vi "J1939 - Tool.vi"() -> ()   [LabVIEW 2019, in "J1939 Workspace Tool.lvlib"]
uses:
  J1939 Workspace Tool.lvlib
  NationalInstruments.VeriStand.SystemStorage
  Workspace Shared/Types/UI.StateVariables.ctl
  <vilib>/NI VeriStand/Display Template Support/DisplayTemplateSupport.llb/enum_Display Template Handler Minimal To Widget Msg.ctl
  <vilib>/NI VeriStand/Execution/Workspace/SystemStateRegEventRef.ctl
  <vilib>/NI VeriStand/Execution/Workspace/Target State Info.ctl
  <vilib>/NI VeriStand/Execution/Workspace/Target State.ctl
  Shared/Types/Private Data.ctl
  <vilib>/NI/STM/TCP/TCP Connection Info.ctl
  <vilib>/NI/STM/SubVIs/MetaDataElement.ctl
  Shared/Types/Error Cluster.ctl
  Shared/Types/Error Types.ctl
  <vilib>/NI VeriStand/Display Template Support/DisplayTemplateSupport.llb/enum_Display Template Handler Minimal To Workspace.ctl
  <vilib>/NI VeriStand/Execution/Workspace/WorkspaceAPI.ctl
  <vilib>/NI VeriStand/Execution/Workspace/SystemStateEventRef.ctl
  Workspace Shared/Types/UI.Refs.ctl
  <vilib>/Utility/miscctls.llb/LVStringsAndValuesArrayTypeDef_U8.ctl
  Shared/J1939 Utilities/SubVIs/Convert CAN Arb ID to J1939 ID.vi
  Shared/J1939 Utilities/J1939 Utilities.lvlib
  Shared/J1939 Addon Shared.lvlib
  <vilib>/NI/STM/NI STM.lvlib
  Workspace Shared/J1939 Workspace Shared.lvlib
  <vilib>/NI VeriStand/Execution/Workspace/NI_VS Workspace ExecutionAPI.lvlib
  NationalInstruments.VeriStand.ClientAPI
panel:
  in  "NIVS.Workspace Event":refnum<event-registration>
  in  "NIVS.Gateway IP Address":string
  in  "NIVS.System Definition Root":refnum<k24>
  in  "Tab Control":enum32{"DTCs", "Custom RQST", "RAW FRAME"}(tab)
  in  "Refresh Continuous":bool
  in  "Clear DTC":bool
  in  "Refresh DTCs":bool
  in  "DTCs":i32(listbox)
  in  "Addresses":string(tree)
  in  "Refresh Addresses":bool
  out "Response":string
  in  "Request":bool
  in  "PGN":u32 format="%.0x"
  in  "DA":u8(ring)
  in  "Clear Array":bool
  in  "RAW":bool
  out "Priority":u8 format="%02x"
  out "SA":u8 format="%02x"
  out "PGN":u32 format="%06x"
  in  "Identifier":u32 format="%08x"
  in  "Data":u8[](array[numeric])=[0, 0, 0, 0, 0, 0, 0, 0] format="%.0x"
  out "Device":string
  in  "Errors":bool
  # "This is the root reference to the active System Definition file. You could use this to read the configuration or populate a tree with channels. You are free to close this reference, but it will be closed for you if you don't."
  # "The SystemStorageUI .NET assembly provides controls to display data configured in the System Definition file."
  # "This is the IP Address of the VeriStand Gateway to which the Workspace is connected. Use this to open all the .NET Manager references. Usually the Gateway is running on localhost, but it could be running on a neighbor's machine."
  # "This registered string User Event is used to help instruct your tool to shut down when the Workspace is closing."
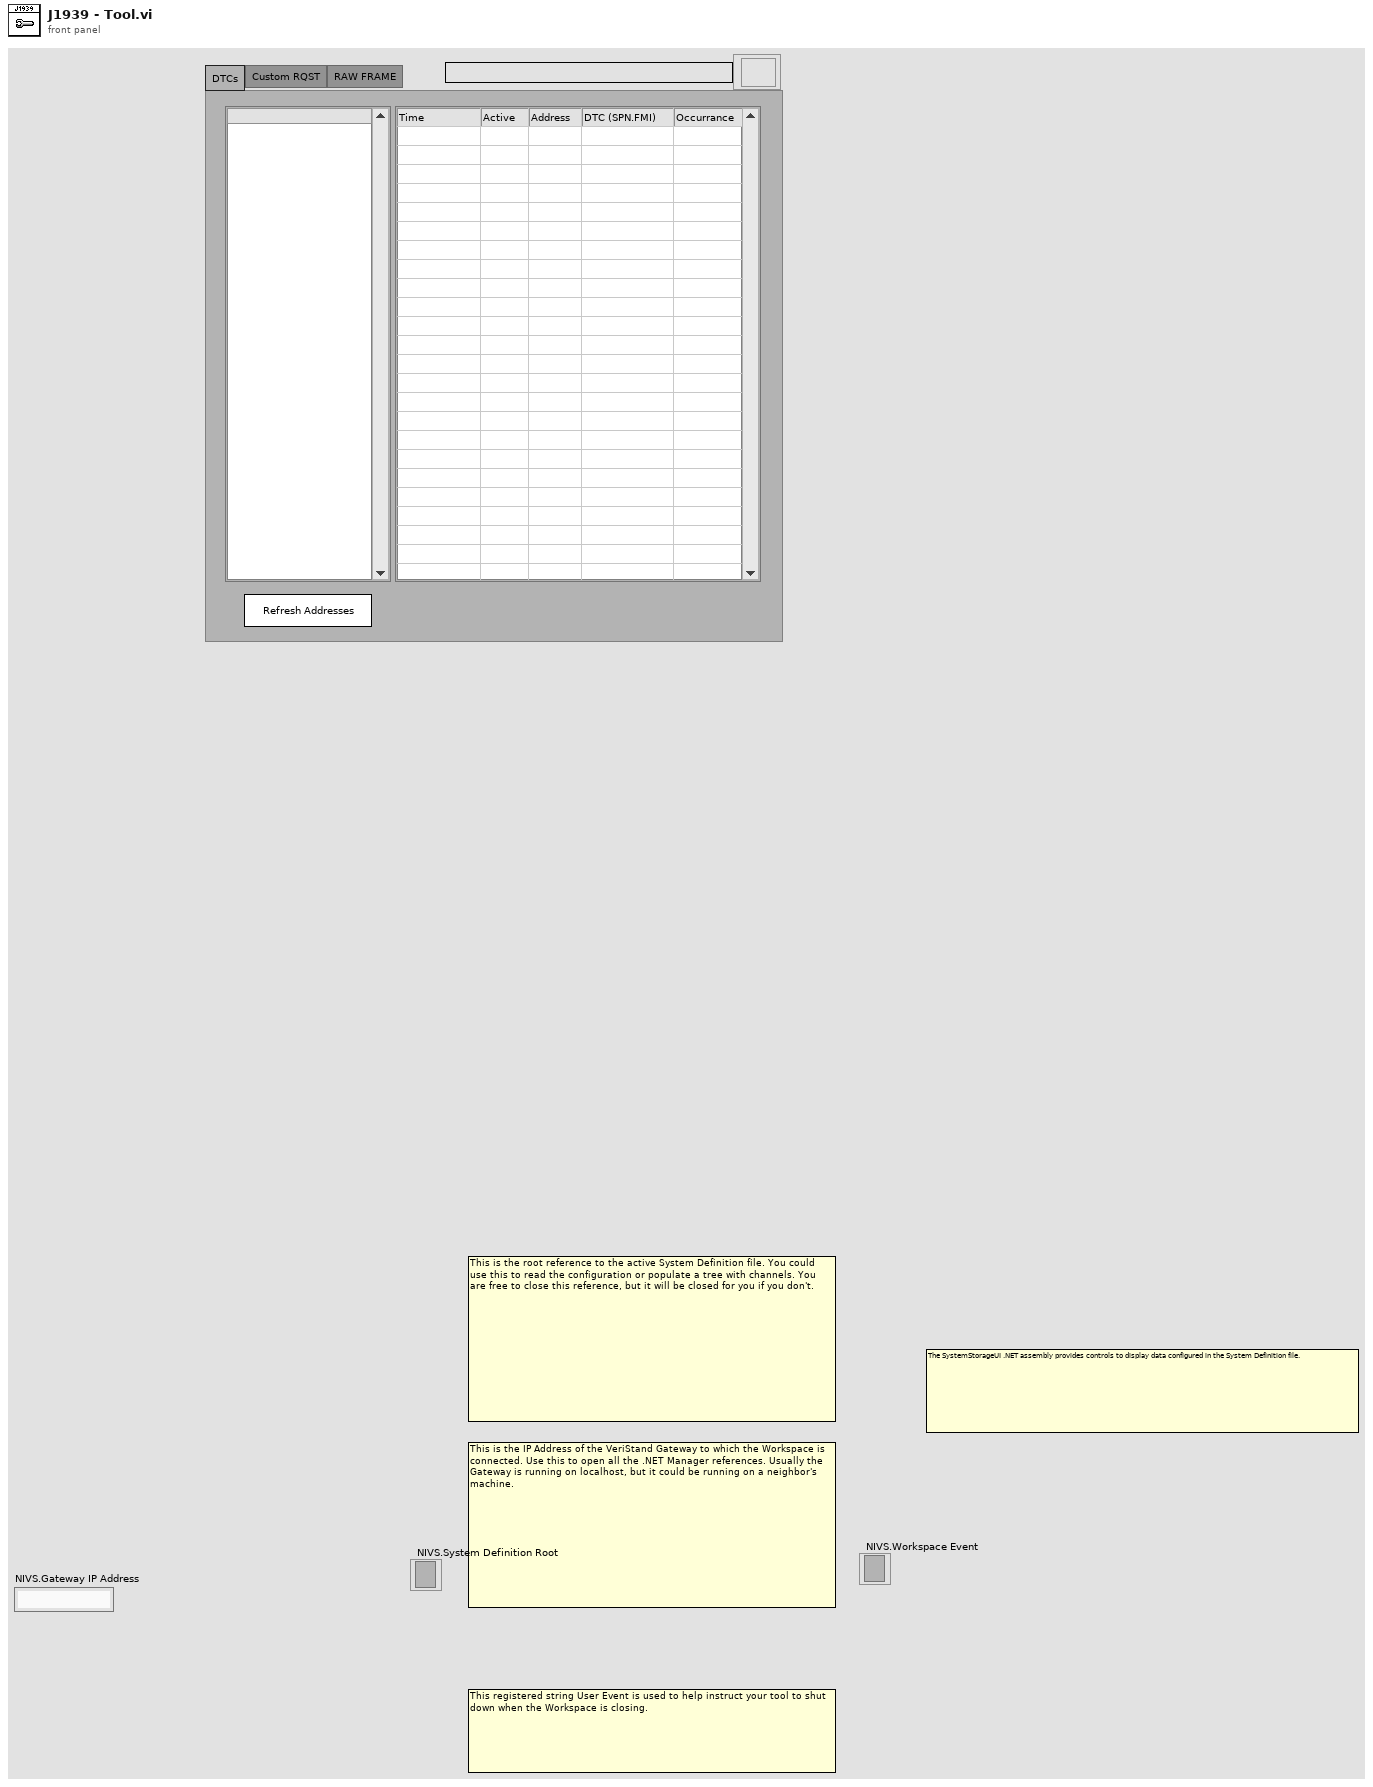
[diagram p1: front panel]
types:
  T1 = typedef "J1939 Addon Shared.lvlib/Private Data.ctl" = cluster{"PGN":u32, "DA":u8, "CD Path":string, "CD IP":string}
  T2 = typedef "J1939 Workspace Shared.lvlib/UI.StateVariables.ctl" = cluster{"NIVS.Gateway IP Address":string, "LaunchConfig.Ref":refnum<user-event>, "Events.Refs":cluster{"LaunchConfig":refnum<event-registration>, "SystemChange":T3, "NIVS.Workspace":refnum<event-registration>}, "State":T1, "TCP.Refs":T4, "Addresses.LUT":variant, "Errors.Q":refnum<queue>, "NIVS.SysDefRoot":refnum<k24>, "State.Notifier":refnum<user-event>, "NIVS.Workspace":T6, "DTCs.Refresh":bool, "NIVS.State.Refs":T7, "UI.Refs":T8, "Addon.Connected":bool, "DTCs.Timer":u32, "Mode.Tool?":bool}
  T3 = typedef "NI_VS Workspace ExecutionAPI.lvlib/SystemStateRegEventRef.ctl" = refnum<event-registration>
  T4 = typedef "NI STM.lvlib/TCP Connection Info.ctl" = cluster{"connection ID":refnum<k5>, "meta data":T5[]}
  T5 = typedef "NI STM.lvlib/MetaDataElement.ctl" = string
  T6 = typedef "NI_VS Workspace ExecutionAPI.lvlib/WorkspaceAPI.ctl" = refnum<k24>
  T7 = typedef "NI_VS Workspace ExecutionAPI.lvlib/SystemStateEventRef.ctl" = cluster{"CustDatRef":refnum<user-event>, "EvtRef":refnum<k27>, "Target State User Event":refnum<user-event>}
  T8 = typedef "J1939 Workspace Shared.lvlib/UI.Refs.ctl" = cluster{"ParentVI":refnum<vi>, "DTCs":refnum<vi>, "Addresses":refnum<vi>, "Device":refnum<vi>, "Data":refnum<vi>, "Identifier":refnum<vi>, "PGN":refnum<vi>, "DA":refnum<vi>, "Refresh Continuous":refnum<vi>, "Errors":refnum<vi>, "Refresh Addresses":refnum<vi>, "Refresh DTCs":refnum<vi>, "Clear DTC":refnum<vi>, "Request":refnum<vi>, "Clear Array":refnum<vi>, "RAW":refnum<vi>, "SA":refnum<vi>, "PGN Ind":refnum<vi>, "Priority":refnum<vi>, "Response":refnum<vi>}
  T9 = enum8{"Enabled", "Disabled", "Disabled and Grayed Out"}
  T10 = typedef "LVStringsAndValuesArrayTypeDef_U8.ctl" = cluster{"String":string, "Value":u8}[]
  T11 = typedef "enum_Display Template Handler Minimal To Workspace.ctl" = cluster{"Operation":enum16{"SetCustomData", "DeleteItem"}, "Data":variant}
  T12 = cluster{"LaunchConfig":refnum<event-registration>, "SystemChange":T3, "NIVS.Workspace":refnum<event-registration>}
  T13 = typedef "enum_Display Template Handler Minimal To Widget Msg.ctl" = enum16{"Stop", "LaunchConfigDialog"}
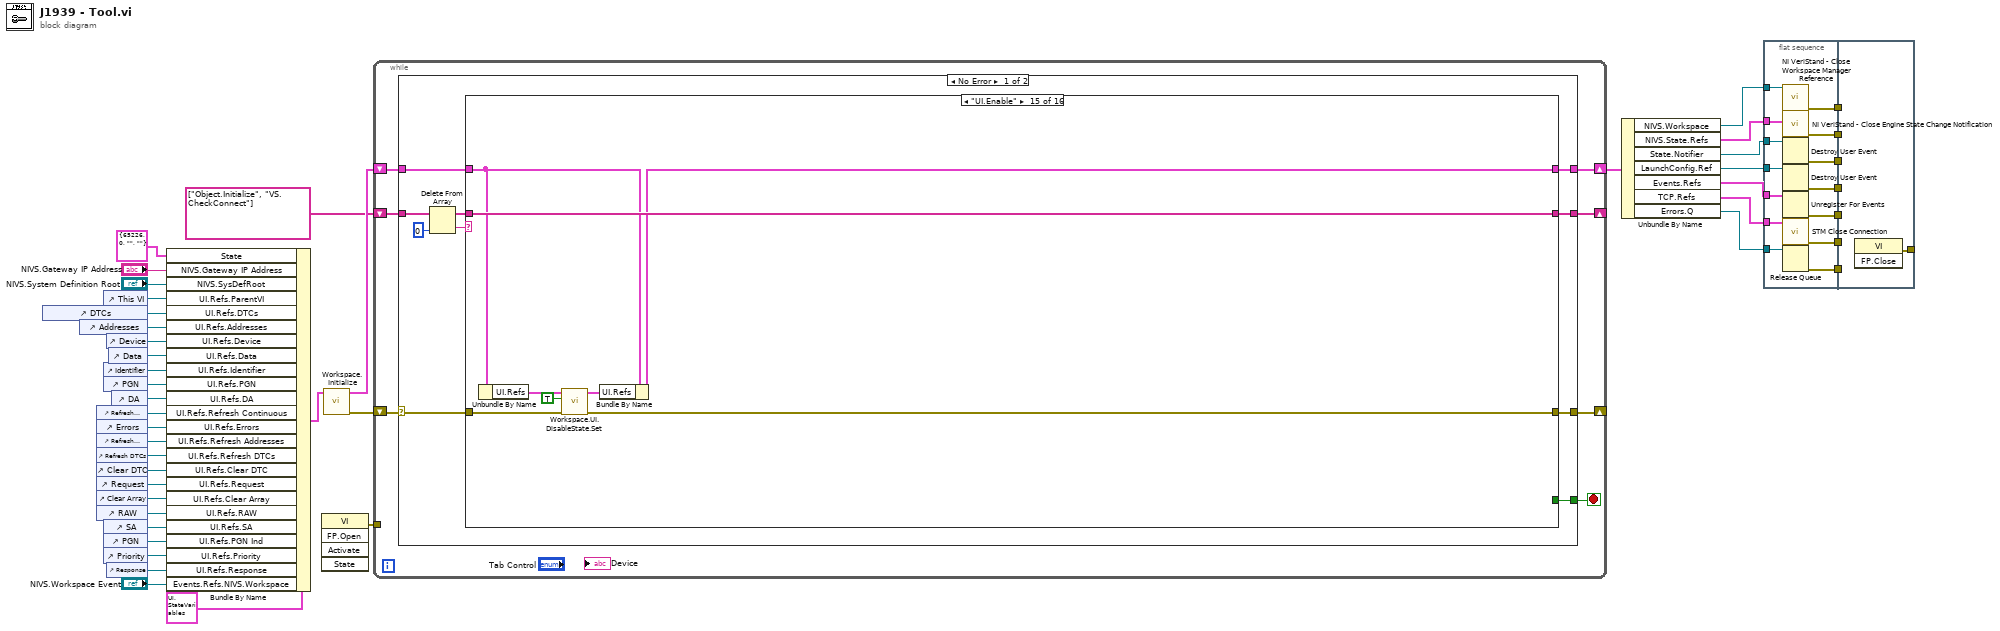
[diagram p0: block diagram]
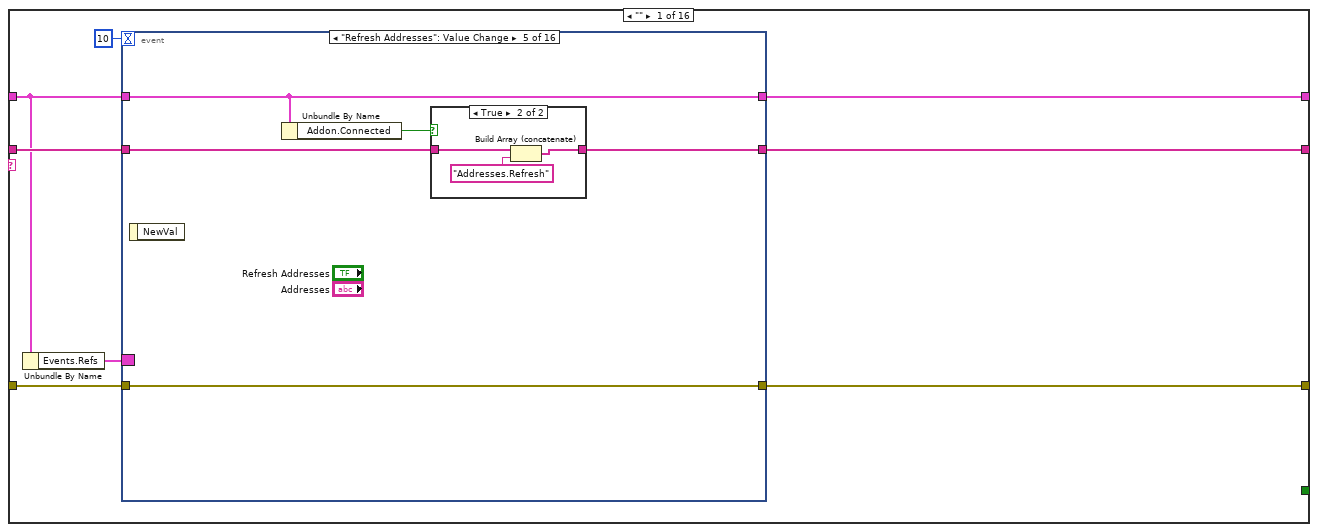
[diagram p2: hidden frame]
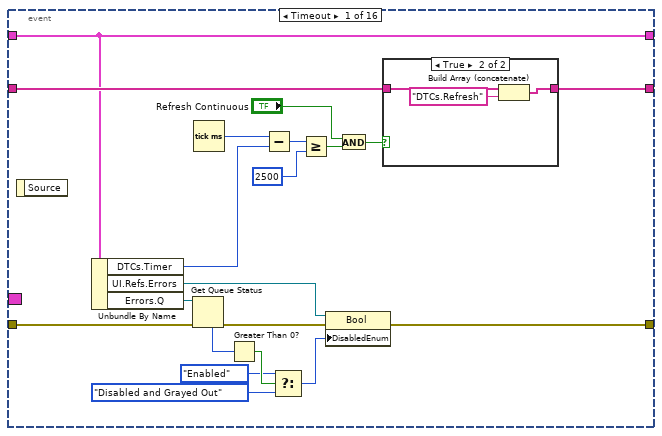
[diagram p3: hidden frame]
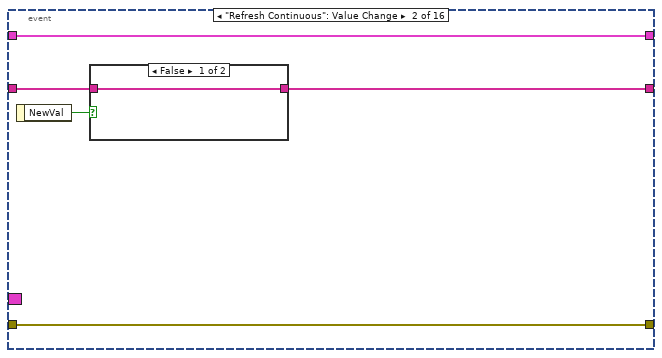
[diagram p5: hidden frame]
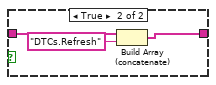
[diagram p6: hidden frame]
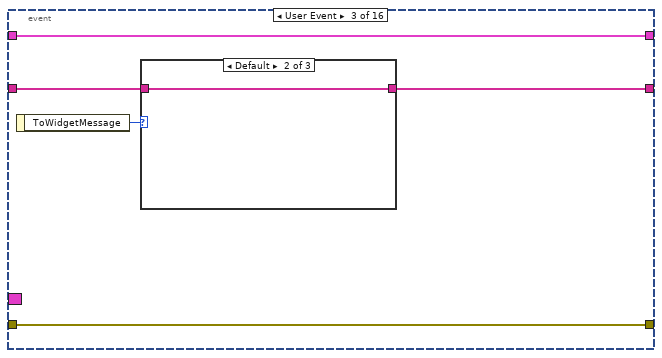
[diagram p7: hidden frame]
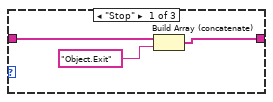
[diagram p8: hidden frame]
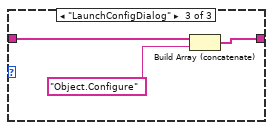
[diagram p9: hidden frame]
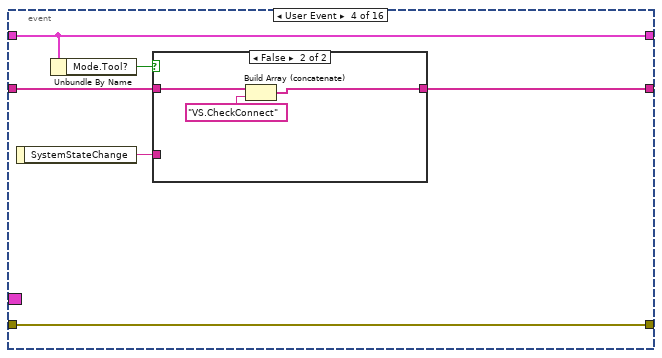
[diagram p10: hidden frame]
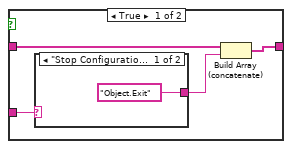
[diagram p11: hidden frame]
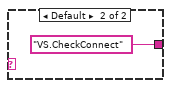
[diagram p12: hidden frame]
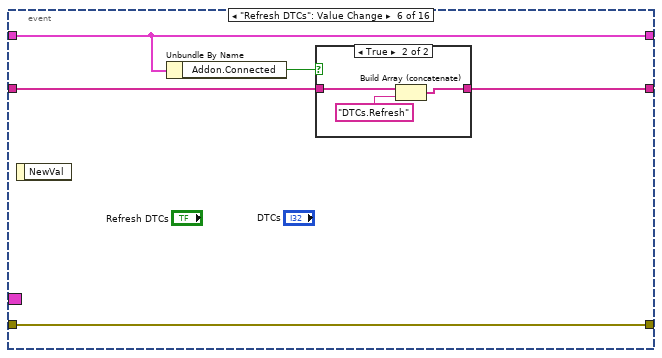
[diagram p14: hidden frame]
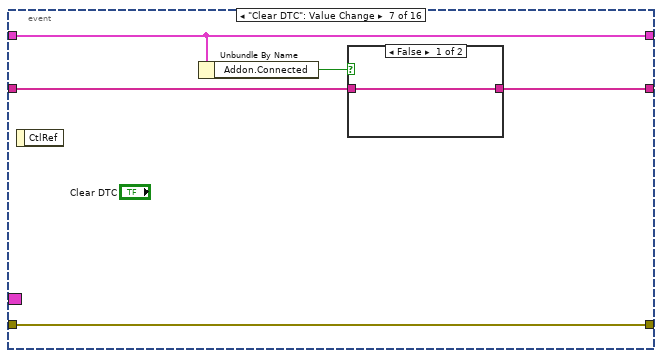
[diagram p16: hidden frame]
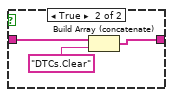
[diagram p17: hidden frame]
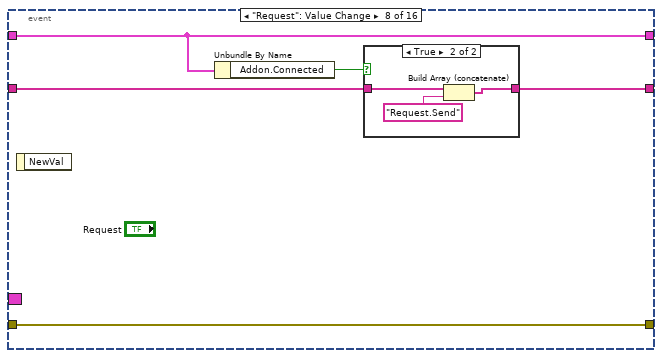
[diagram p18: hidden frame]
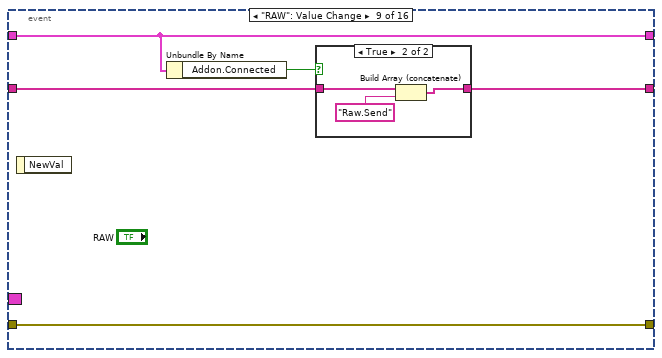
[diagram p20: hidden frame]
diagram:
  n1 = control-ref of="DTCs"() -> (w39:refnum<vi>)
  n2 = control-ref of="Addresses"() -> (w38:refnum<vi>)
  n3 = control-ref of="Refresh Continuous"() -> (w32:refnum<vi>)
  n4 = control-ref of="Errors"() -> (w31:refnum<vi>)
  n5 = control-ref of="Refresh Addresses"() -> (w30:refnum<vi>)
  n6 = control-ref of="Refresh DTCs"() -> (w29:refnum<vi>)
  n7 = control-ref of="Clear DTC"() -> (w28:refnum<vi>)
  n8 = control-ref of="Request"() -> (w27:refnum<vi>)
  n9 = control-ref of="Clear Array"() -> (w26:refnum<vi>)
  n10 = control-ref of="RAW"() -> (w25:refnum<vi>)
  n11 = control-ref of="This VI"() -> (w40:refnum<vi>)
  n12 = control-ref of="Identifier"() -> (w35:refnum<vi>)
  n13 = control-ref of="PGN"() -> (w34:refnum<vi>)
  n14 = control-ref of="SA"() -> (w4:refnum<vi>)
  n15 = control-ref of="PGN"() -> (w3:refnum<vi>)
  n16 = control-ref of="Priority"() -> (w2:refnum<vi>)
  n17 = control-ref of="Device"() -> (w37:refnum<vi>)
  n18 = control-ref of="Response"() -> (w1:refnum<vi>)
  n19 = control-ref of="Data"() -> (w36:refnum<vi>)
  n20 = control-ref of="DA"() -> (w33:refnum<vi>)
  n21 = Bundle By Name(cluster=T2 {"NIVS.Gateway IP Address"="", "LaunchConfig.Ref"=refnum, "Events.Refs"={"LaunchConfig"=refnum, "SystemChange"=refnum, "NIVS.Workspace"=refnum}, "State"={"PGN"=0, "DA"=0, "CD Path"="", "CD IP"=""}, "TCP.Refs"={"connection ID"=refnum, "meta data"=[]}, "Addresses.LUT"=variant, "Errors.Q"=refnum, "NIVS.SysDefRoot"=refnum, "State.Notifier"=refnum, "NIVS.Workspace"=refnum, "DTCs.Refresh"=FALSE, "NIVS.State.Refs"={"CustDatRef"=refnum, "EvtRef"=refnum, "Target State User Event"=refnum}, "UI.Refs"={"ParentVI"=refnum, "DTCs"=refnum, "Addresses"=refnum, "Device"=refnum, "Data"=refnum, "Identifier"=refnum, "PGN"=refnum, "DA"=refnum, "Refresh Continuous"=refnum, "Errors"=refnum, "Refresh Addresses"=refnum, "Refresh DTCs"=refnum, "Clear DTC"=refnum, "Request"=refnum, "Clear Array"=refnum, "RAW"=refnum, "SA"=refnum, "PGN Ind"=refnum, "Priority"=refnum, "Response"=refnum}, "Addon.Connected"=FALSE, "DTCs.Timer"=0, "Mode.Tool?"=FALSE}, "State"=T1 {"PGN"=65226, "DA"=0, "CD Path"="", "CD IP"=""} ("Cluster"), "NIVS.Gateway IP Address"="NIVS.Gateway IP Address", "NIVS.SysDefRoot"="NIVS.System Definition Root", "UI.Refs.ParentVI"=w40, "UI.Refs.DTCs"=w39, "UI.Refs.Addresses"=w38, "UI.Refs.Device"=w37, "UI.Refs.Data"=w36, "UI.Refs.Identifier"=w35, "UI.Refs.PGN"=w34, "UI.Refs.DA"=w33, "UI.Refs.Refresh Continuous"=w32, "UI.Refs.Errors"=w31, "UI.Refs.Refresh Addresses"=w30, "UI.Refs.Refresh DTCs"=w29, "UI.Refs.Clear DTC"=w28, "UI.Refs.Request"=w27, "UI.Refs.Clear Array"=w26, "UI.Refs.RAW"=w25, "UI.Refs.SA"=w4, "UI.Refs.PGN Ind"=w3, "UI.Refs.Priority"=w2, "UI.Refs.Response"=w1, "Events.Refs.NIVS.Workspace"="NIVS.Workspace Event") -> (w42:T2)
  n22 = invoke class="VI" method="FP.Open"() -> (error out=w12:errorcluster)  [unwired: 5 in, 4 out]
  n23 = call "Workspace.Initialize.vi"("State"=w42) -> ("error out"=w41:errorcluster, "State"=w24:T2)  [unwired: 9 in]
  n24 = while {
    shift-right: [w50] -> _
    shift-left: w41 -> [w51]
    shift-right: [w46] -> w22
    shift-left: w24 -> [w49]
    shift-right: [w47] -> _
    shift-left: string[] ["Object.Initialize", "VS.CheckConnect"] -> [w48]
    tunnel: w12 -> [_]
    stop <- w52 stop-if-true
    n25 = case shown="No Error" w51 {
      selector: w51 -> [w53 w461]
      tunnel: [w62 FALSE] -> w52
      tunnel: [w54 w459] -> w50
      tunnel: w49 -> [w61 w456]
      tunnel: w48 -> [w59 w457]
      tunnel: [w56 w457] -> w47
      tunnel: [w55 w456] -> w46
      frame No Error {
        n26 = Delete From Array(array=w59, index=0) -> (deleted portion=w58:string, array with subset deleted=w57:string[])  [unwired: 1 in]
        n27 = case shown="\"UI.Enable\"" w58 {
          selector: w58 -> [_ _ _ _ _ _ _ _ _ _ _ _ _ _ _ w451]
          tunnel: [_ _ _ _ _ _ _ _ TRUE _ _ _ _ _ _ _] -> w62
          tunnel: w61 -> [w64 w227 w236 w253 w306 w311 w345 w373 w376 w381 w405 w413 w425 w434 w442 w454]
          tunnel: w57 -> [w68 w234 w246 w262 w307 w309 w351 w369 w377 w379 w406 w414 w421 w441 w449 w455]
          tunnel: [w69 w234 w246 w262 w307 w308 w350 w369 w377 w378 w406 w414 w421 w441 w449 w455] -> w56
          tunnel: [w67 w224 w235 w263 w306 w310 w344 w372 w376 w382 w405 w412 w422 w435 w443 w454] -> w55
          tunnel: [w66 w223 w245 w248 w283 w314 w347 w368 w375 w390 w401 w407 w420 w436 w444 w453] -> w54
          tunnel: w53 -> [w65 w223 w245 w249 w280 w315 w346 w368 w375 w391 w400 w407 w420 w437 w445 w453]
          frame "" {
            n28 = Unbundle By Name(w64) -> ("Events.Refs"=w63:T12)
            n29 = event shown="[4] \"Refresh Addresses\": Value Change" {
              selector: w63 -> [_ _ _ _ _ _ _ _ _ _ _ _ _ _ _ _]
              dyn-events: _ -> [_ _ _ _ _ _ _ _ _ _ _ _ _ _ _ _]
              timeout: 10 -> [_ _ _ _ _ _ _ _ _ _ _ _ _ _ _ _]
              tunnel: w64 -> [w79 w98 w108 w117 w134 w142 w149 w160 w169 w178 w187 w191 w198 w208 w213 w222]
              tunnel: [w80 w96 w104 w120 w132 w140 w150 w158 w167 w176 w186 w192 w200 w204 w210 w219] -> w69
              tunnel: w68 -> [w81 w97 w105 w121 w133 w141 w151 w159 w168 w177 w189 w192 w200 w205 w211 w220]
              tunnel: [w79 w98 w108 w117 w134 w142 w149 w160 w169 w178 w187 w191 w198 w208 w213 w222] -> w67
              tunnel: [w73 w99 w107 w118 w135 w144 w153 w162 w171 w180 w188 w190 w199 w207 w212 w221] -> w66
              tunnel: w65 -> [w75 w99 w107 w118 w135 w144 w153 w162 w171 w180 w188 w190 w199 w207 w212 w221]
              event Timeout {
                n30 = event-data() -> ()  [unwired: 2 out]
                n31 = Unbundle By Name(w79) -> ("DTCs.Timer"=w72:u32, "UI.Refs.Errors"=w77:refnum<vi>, "Errors.Q"=w78:refnum<queue>)
                n32 = Get Queue Status(queue=w78, error in (no error)=w75) -> (error out=w76:errorcluster, # elements in queue=w90:i32)  [unwired: 1 in, 6 out]
                n33 = Tick Count (ms)() -> (millisecond timer value=w84:u32)
                n34 = Greater Than 0?(x=w90) -> (x > 0?=w89:bool)
                n35 = Subtract(x=w84, y=w72) -> (x-y=w86:u32)
                n36 = Select(t=T9."Enabled" ("Disabled"), s=w89, f=T9."Disabled and Grayed Out") -> (s? t:f=w74:T9)
                n37 = Greater Or Equal?(x=w86, y=u32 2500) -> (x >= y?=w71:bool)
                n38 = property class="Bool"(reference=w77, error in=w76, "DisabledEnum"=w74) -> (error out=w73:errorcluster)  [unwired: 1 out]
                n39 = And(x="Refresh Continuous", y=w71) -> (x .and. y?=w82:bool)
                n40 = case shown="True" w82 {
                  tunnel: w81 -> [w91 w93]
                  tunnel: [w91 w92] -> w80
                  frame False {
                  }
                  frame True {
                    n41 = Build Array (concatenate)(w93, "DTCs.Refresh" ("NewVal")) -> (w92:string[])
                  }
                }
              }
              event "Refresh Continuous": Value Change {
                n42 = event-data() -> ("NewVal"=w95:bool)  [unwired: 1 out]
                n43 = case shown="False" w95 {
                  tunnel: w97 -> [w100 w102]
                  tunnel: [w100 w101] -> w96
                  frame False {
                  }
                  frame True {
                    n44 = Build Array (concatenate)(w102, "DTCs.Refresh" ("NewVal")) -> (w101:string[])
                  }
                }
              }
              event User Event {
                n45 = event-data() -> ("ToWidgetMessage"=w106:T13)  [unwired: 1 out]
                n46 = case shown="Default" w106 {
                  tunnel: w105 -> [w111 w112 w115]
                  tunnel: [w110 w112 w114] -> w104
                  frame "Stop" {
                    n47 = Build Array (concatenate)(w111, "Object.Exit") -> (w110:string[])
                  }
                  frame Default {
                  }
                  frame "LaunchConfigDialog" {
                    n48 = Build Array (concatenate)(w115, "Object.Configure") -> (w114:string[])
                  }
                }
              }
              event User Event {
                n49 = event-data() -> ("SystemStateChange"=w116:string)  [unwired: 1 out]
                n50 = Unbundle By Name(w117) -> ("Mode.Tool?"=w119:bool)
                n51 = case shown="False" w119 {
                  tunnel: w121 -> [w125 w130]
                  tunnel: [w124 w129] -> w120
                  tunnel: w116 -> [w123 _]
                  frame True {
                    # "System state not connected"
                    n52 = case shown="\"Stop Configuration\"" w123 {
                      tunnel: ["Object.Exit" "VS.CheckConnect"] -> w122
                      frame "Stop Configuration" {
                      }
                      frame Default {
                      }
                    }
                    n53 = Build Array (concatenate)(w125, w122) -> (w124:string[])
                  }
                  frame False {
                    # "System state is connected"
                    n54 = Build Array (concatenate)(w130, "VS.CheckConnect") -> (w129:string[])
                  }
                }
              }
              event "Refresh Addresses": Value Change {
                n55 = event-data() -> ()  [unwired: 2 out]
                n56 = Unbundle By Name(w134) -> ("Addon.Connected"=w131:bool)
                n57 = case shown="True" w131 {
                  tunnel: w133 -> [w136 w138]
                  tunnel: [w136 w137] -> w132
                  frame False {
                  }
                  frame True {
                    n58 = Build Array (concatenate)(w138, "Addresses.Refresh") -> (w137:string[])
                  }
                }
              }
              event "Refresh DTCs": Value Change {
                n59 = event-data() -> ()  [unwired: 2 out]
                n60 = Unbundle By Name(w142) -> ("Addon.Connected"=w143:bool)
                n61 = case shown="True" w143 {
                  tunnel: w141 -> [w145 w147]
                  tunnel: [w145 w146] -> w140
                  frame False {
                  }
                  frame True {
                    n62 = Build Array (concatenate)(w147, "DTCs.Refresh") -> (w146:string[])
                  }
                }
              }
              event "Clear DTC": Value Change {
                n63 = event-data() -> ()  [unwired: 2 out]
                n64 = Unbundle By Name(w149) -> ("Addon.Connected"=w152:bool)
                n65 = case shown="False" w152 {
                  tunnel: w151 -> [w154 w156]
                  tunnel: [w154 w155] -> w150
                  frame False {
                  }
                  frame True {
                    n66 = Build Array (concatenate)(w156, "DTCs.Clear") -> (w155:string[])
                  }
                }
              }
              event "Request": Value Change {
                n67 = event-data() -> ()  [unwired: 2 out]
                n68 = Unbundle By Name(w160) -> ("Addon.Connected"=w161:bool)
                n69 = case shown="True" w161 {
                  tunnel: w159 -> [w163 w165]
                  tunnel: [w163 w164] -> w158
                  frame False {
                  }
                  frame True {
                    n70 = Build Array (concatenate)(w165, "Request.Send") -> (w164:string[])
                  }
                }
              }
              event "RAW": Value Change {
                n71 = event-data() -> ()  [unwired: 2 out]
                n72 = Unbundle By Name(w169) -> ("Addon.Connected"=w170:bool)
                n73 = case shown="True" w170 {
                  tunnel: w168 -> [w172 w174]
                  tunnel: [w172 w173] -> w167
                  frame False {
                  }
                  frame True {
                    n74 = Build Array (concatenate)(w174, "Raw.Send") -> (w173:string[])
                  }
                }
              }
              event "Clear Array": Value Change {
                n75 = event-data() -> ()  [unwired: 2 out]
                n76 = Unbundle By Name(w178) -> ("Addon.Connected"=w179:bool)
                n77 = case shown="True" w179 {
                  tunnel: w177 -> [w181 w183]
                  tunnel: [w181 w182] -> w176
                  frame False {
                  }
                  frame True {
                    n78 = Build Array (concatenate)(w183, "Raw.Clear") -> (w182:string[])
                  }
                }
              }
              event "Addresses": Value Change {
                n79 = event-data() -> ()  [unwired: 2 out]
                n80 = Build Array (concatenate)(w189, "DTCs.Refresh" ("NewVal")) -> (w186:string[])
              }
              event "Identifier": Value Change {
                n81 = event-data() -> ("NewVal"=w193:u32)  [unwired: 1 out]
                n82 = call-poly "Common Conversions.vi"("Arb ID"=w193) -> ("Priority"=→"Priority":u8, "PGN"=→"PGN":u32, "Source Address"=→"SA":u8)  [unwired: 11 in, 1 out]
              }
              event "Errors": Value Change {
                n83 = event-data() -> ()  [unwired: 2 out]
                n84 = Unbundle By Name(w198) -> ("Errors.Q"=w197:refnum<queue>)
                n85 = flat-sequence {
                  tunnel: [w202] -> w201
                  tunnel: w197 -> [w202]
                  frame #0 {
                  }
                }
                n86 = call "Error Display.vi"("queue out"=w201) -> ()  [unwired: 11 in]
              }
              event Panel Close? {
                n87 = event-data() -> ()  [unwired: 5 out]
                n88 = Build Array (concatenate)(w205, "Object.Exit") -> (w204:string[])
                n89 = event-data("Discard?"=TRUE) -> ()  [unwired: 1 in, 1 out]
              }
              event User Event {
                n90 = event-data() -> ("Workspace Event"=w209:string)  [unwired: 1 out]
                n91 = case shown="\"Disconnect\", \"Shut Down\"" w209 {
                  tunnel: w211 -> [w214 w217]
                  tunnel: [w214 w216] -> w210
                  frame Default {
                  }
                  frame "Disconnect", "Shut Down" {
                    n92 = Build Array (concatenate)(w217, "Object.Exit") -> (w216:string[])
                  }
                }
              }
              event Menu Selection (User) {
                n93 = event-data() -> ("ItemTag"=w218:string)  [unwired: 1 out]
                n94 = Build Array (concatenate)(w220, w218) -> (w219:string[])
              }
            }
          }
          frame "Addresses.Refresh" {
            n95 = Unbundle By Name(w227) -> ("UI.Refs.Addresses"=w233:refnum<vi>, "UI.Refs.DA"=w232:refnum<vi>, "TCP.Refs"=w231:T4, "State"=w230:T1, "Errors.Q"=w229:refnum<queue>, "UI.Refs.ParentVI"=w228:refnum<vi>)
            n96 = call "Request Addresses Event.vi"("connection info"=w231, "DA"=w232, "Addresses"=w233, "State Variables"=w230, "Error Q"=w229, "VI Ref"=w228) -> ("connection info"=w226:T4, "Address Lookup Table Out"=w225:variant)  [unwired: 8 in]
            n97 = Bundle By Name(cluster=w227, "TCP.Refs"=w226, "Addresses.LUT"=w225) -> (w224:T2)
          }
          frame "DTCs.Clear" {
            n98 = Unbundle By Name(w236) -> ("UI.Refs.Addresses"=w239:refnum<vi>, "TCP.Refs"=w244:T4, "State"=w243:T1, "Addresses.LUT"=w242:variant, "Errors.Q"=w241:refnum<queue>, "UI.Refs.ParentVI"=w240:refnum<vi>)
            n99 = call "Clear DTCs Event.vi"("connection info"=w244, "Addresses"=w239, "State Variables"=w243, "Address Lookup Table"=w242, "Error Q"=w241, "VI Ref"=w240) -> ("connection info"=w238:T4, "Address Lookup Table Out"=w237:variant)  [unwired: 8 in]
            n100 = Bundle By Name(cluster=w236, "TCP.Refs"=w238, "Addresses.LUT"=w237) -> (w235:T2)
          }
          frame "DTCs.Refresh" {
            n101 = Unbundle By Name(w253) -> ("UI.Refs.DTCs"=w260:refnum<vi>, "UI.Refs.Addresses"=w259:refnum<vi>, "TCP.Refs"=w258:T4, "State"=w257:T1, "Addresses.LUT"=w256:variant, "Errors.Q"=w255:refnum<queue>, "UI.Refs.ParentVI"=w254:refnum<vi>, "UI.Refs.Refresh Continuous"=w250:refnum<vi>)
            n102 = property class="Bool (strict)"(reference=w250, error in=w249) -> (error out=w248:errorcluster, "Value"=w247:bool)  [unwired: 1 out]
            n103 = Not(x=w247) -> (.not. x?=w261:bool)
            n104 = flat-sequence {
              tunnel: w256 -> [w276]
              tunnel: w258 -> [w274]
              tunnel: w257 -> [w272]
              tunnel: w261 -> [w271]
              tunnel: [w275] -> w266
              tunnel: [w273] -> w265
              tunnel: w260 -> [w270]
              tunnel: w259 -> [w269]
              tunnel: w255 -> [w268]
              tunnel: w254 -> [w267]
              tunnel: [w278] -> w251
              tunnel: [w279] -> w252
              tunnel: w266 -> [w279]
              tunnel: w265 -> [w278]
              tunnel: [w277] -> w264
              frame #0 {
                n105 = call "Refresh DTCs Event.vi"("connection info"=w274, "Addresses"=w269, "DTCs"=w270, "State Variables"=w272, "Address Lookup Table"=w276, "To Top (T)"=w271, "Error Q"=w268, "VI Ref"=w267) -> ("connection info"=w273:T4, "Address Lookup Table Out"=w275:variant)  [unwired: 6 in]
              }
              frame #1 {
                n106 = Tick Count (ms)() -> (millisecond timer value=w277:u32)
              }
            }
            n107 = Bundle By Name(cluster=w253, "DTCs.Timer"=w264, "TCP.Refs"=w251, "Addresses.LUT"=w252) -> (w263:T2)
          }
          frame "Object.Initialize" {
            n108 = Unbundle By Name(w306) -> ("UI.Refs.Errors"=w281:refnum<vi>, "UI.Refs.Data"=w288:refnum<vi>, "UI.Refs.Identifier"=w292:refnum<vi>, "UI.Refs.DA"=w294:refnum<vi>, "UI.Refs.PGN"=w297:refnum<vi>, "UI.Refs.DTCs"=w300:refnum<vi>, "UI.Refs.Addresses"=w303:refnum<vi>, "UI.Refs.Refresh Continuous"=w304:refnum<vi>)
            n109 = property class="Bool (strict)"(reference=w304, error in=w280, "Value"=FALSE) -> (error out=w301:errorcluster)  [unwired: 1 out]
            n110 = invoke class="Tree (strict)" method="Edit Tree Items.Delete"(reference=w303, error in=w301, "Delete Children"=TRUE ("Delete Children?")) -> (error out=w298:errorcluster)  [unwired: 2 in, 4 out]
            n111 = property class="MCListbox (strict)"(reference=w300, error in=w298, "ItemNames"=string[][] [] ("Item Names")) -> (error out=w295:errorcluster)  [unwired: 1 out]
            n112 = property class="DigNum (strict)"(reference=w297, error in=w295, "Value"=u32 0) -> (error out=w293:errorcluster)  [unwired: 1 out]
            n113 = property class="Ring (strict)"(reference=w294, error in=w293, "Value"=u8 0, "StringsAndValues[]"=T10 [] ("Strings And Values []")) -> (error out=w291:errorcluster)  [unwired: 1 out]
            n114 = property class="DigNum (strict)"(reference=w292, error in=w291, "Val(Sgnl)"=u32 0 ("Value (Signaling)")) -> (error out=w287:errorcluster)  [unwired: 1 out]
            n115 = property class="Arr (strict)"(reference=w288, error in=w287, "Value"=u8[] []) -> (error out=w284:errorcluster)  [unwired: 1 out]
            n116 = property class="Bool"(reference=w281, error in=w284, "DisabledEnum"=T9."Disabled and Grayed Out" ("f")) -> (error out=w283:errorcluster)  [unwired: 1 out]
          }
          frame "Object.Configure" {
            n117 = Unbundle By Name(w311) -> ("State"=w313:T1, "State.Notifier"=w316:refnum<user-event>, "NIVS.SysDefRoot"=w317:refnum<k24>, "State.CD Path"=w320:string)
            n118 = call "Select Custom Device.vi"("CD Path"=w320, "NIVS.System Definition Root"=w317) -> ("Cancelled?"=w318:bool, "IP Address"=w321:string, "Custom Device Path Out"=w319:string)  [unwired: 7 in]
            n119 = case shown="True" w318 {
              tunnel: w316 -> [w323 _]
              tunnel: w321 -> [w329 _]
              tunnel: w319 -> [w330 _]
              tunnel: w315 -> [w327 w341]
              tunnel: [w327 w341] -> w314
              tunnel: w313 -> [w328 w340]
              tunnel: [w322 w340] -> w312
              tunnel: w309 -> [w326 w339]
              tunnel: [w324 w339] -> w308
              frame False {
                n120 = flat-sequence {
                  tunnel: w330 -> [w338]
                  tunnel: w329 -> [w337]
                  tunnel: w328 -> [w336]
                  tunnel: w323 -> [w333]
                  tunnel: [w332] -> w322
                  tunnel: [w331] -> _
                  frame #0 {
                    n121 = Bundle By Name(cluster=w336, "CD Path"=w338, "CD IP"=w337) -> (w332:T1)
                    n122 = Bundle By Name(cluster=T11 {"Operation"=enum."SetCustomData", "Data"=variant} ("event data"), "Data"=w332) -> (w334:T11)
                    n123 = Generate User Event(user event=w333, event data cluster=w334) -> (error out=w331:errorcluster)  [unwired: 2 in, 1 out]
                  }
                }
                n124 = Build Array (concatenate)(w326, "VS.CheckConnect") -> (w324:string[])
              }
              frame True {
              }
            }
            n125 = Bundle By Name(cluster=w311, "State"=w312) -> (w310:T2)
          }
          frame "Object.Connected" {
            n126 = Unbundle By Name(w345) -> ("TCP.Refs"=w343:T4, "State.CD IP"=w348:string, "State.CD Path"=w349:string)
            n127 = call "STM Close Connection.vi"("connection info"=w343) -> ("error out"=w342:errorcluster)  [unwired: 10 in]
            n128 = flat-sequence {
              tunnel: w351 -> [w363]
              tunnel: [w361] -> w350
              tunnel: w349 -> [w353]
              tunnel: w348 -> [w360]
              tunnel: [w358] -> w347
              tunnel: w346 -> [w357]
              tunnel: w345 -> [w355]
              tunnel: [w354] -> w344
              tunnel: w342 -> [_]
              frame #0 {
                n129 = call "UI.Addon.Path.Parse.vi"("Cached Addon Path"=w353) -> ("Addon Name"=w352:string)  [unwired: 6 in, 4 out]
                n130 = call "Open Connection to Target.vi"("error in (no error)"=w357, "IP Address"=w360, "TCP Service"=w352) -> ("error out"=w359:errorcluster, "connection info"=w356:T4)  [unwired: 7 in]
                n131 = Bundle By Name(cluster=w355, "TCP.Refs"=w356) -> (w354:T2)
                n132 = case shown="No Error" w359 {
                  selector: w359 -> [w364 w367]
                  tunnel: [string[] ["Object.Initialize", "UI.Enable"] ("element") string[] ["Object.Initialize", "UI.Disable"] ("element")] -> w362
                  tunnel: [w364 w367] -> w358
                  frame No Error {
                  }
                  frame Error {
                  }
                }
                n133 = Build Array (concatenate)(w363, w362) -> (w361:string[])
              }
            }
          }
          frame "Object.Disconnected" {
            n134 = Unbundle By Name(w373) -> ("TCP.Refs"=w371:T4)
            n135 = Bundle By Name(cluster=w373, "TCP.Refs"=T4 {"connection ID"=refnum, "meta data"=[]}) -> (w372:T2)
            n136 = call "STM Close Connection.vi"("connection info"=w371) -> ()  [unwired: 10 in, 1 out]
          }
          frame "Object.Exit" {
          }
          frame "VS.CheckConnect" {
            n137 = Unbundle By Name(w381) -> ("UI.Refs.Device"=w388:refnum<vi>, "NIVS.Workspace"=w386:T6, "NIVS.SysDefRoot"=w387:refnum<k24>, "State.CD Path"=w385:string)
            n138 = Current VI's Menubar() -> (w389:refnum<k9>)
            n139 = call "UI.Connection.State.Get.vi"("Menu Ref"=w389, "Name Ref"=w388, "error in (no error)"=w391, "Addon Path in"=w385, "NIVS.System Definition Root in"=w387, "NIVS.Workspace Ref in"=w386) -> ("error out"=w390:errorcluster, "Addon Connected?"=w380:bool, "NIVS.System Definition Root out"=w383:refnum<k24>, "NIVS.Workspace Ref out"=w384:T6)  [unwired: 2 in]
            n140 = case shown="False" w380 {
              tunnel: w379 -> [w394 w397]
              tunnel: [w393 w396] -> w378
              frame False {
                n141 = Build Array (concatenate)(w394, string[] ["Object.Disconnected", "Object.Initialize", "UI.Disable"]) -> (w393:string[])
              }
              frame True {
                n142 = Build Array (concatenate)(w397, "Object.Connected") -> (w396:string[])
              }
            }
            n143 = Bundle By Name(cluster=w381, "NIVS.Workspace"=w384, "NIVS.SysDefRoot"=w383, "Addon.Connected"=w380) -> (w382:T2)
          }
          frame "Raw.Clear" {
            n144 = Unbundle By Name(w405) -> ("UI.Refs.Identifier"=w403:refnum<vi>, "UI.Refs.Data"=w404:refnum<vi>)
            n145 = property class="Arr (strict)"(reference=w404, error in=w400, "Value"=u8[] []) -> (error out=w402:errorcluster)  [unwired: 1 out]
            n146 = property class="DigNum (strict)"(reference=w403, error in=w402, "Val(Sgnl)"=u32 0 ("Value (Signaling)")) -> (error out=w401:errorcluster)  [unwired: 1 out]
          }
          frame "Raw.Send" {
            n147 = Unbundle By Name(w413) -> ("TCP.Refs"=w417:T4, "State"=w416:T1, "Addresses.LUT"=w415:variant, "Errors.Q"=w411:refnum<queue>, "UI.Refs.ParentVI"=w410:refnum<vi>)
            n148 = call "RAW Event.vi"("connection info"=w417, "State Variables"=w416, "Address Lookup Table"=w415, "Identifier"="Identifier", "Data"="Data", "Error Q"=w411, "VI Ref"=w410) -> ("connection info"=w409:T4, "Address Lookup Table Out"=w408:variant)  [unwired: 7 in]
            n149 = Bundle By Name(cluster=w413, "TCP.Refs"=w409, "Addresses.LUT"=w408) -> (w412:T2)
          }
          frame "Request.Send" {
            n150 = Unbundle By Name(w425) -> ("TCP.Refs"=w430:T4, "State"=w429:T1, "Addresses.LUT"=w428:variant, "Errors.Q"=w427:refnum<queue>, "UI.Refs.ParentVI"=w426:refnum<vi>)
            n151 = call "Request Event.vi"("connection info"=w430, "State Variables"=w429, "Address Lookup Table"=w428, "PGN"="PGN", "DA"="DA", "Error Q"=w427, "VI Ref"=w426) -> ("connection info"=w424:T4, "Response"=→"Response":string, "Address Lookup Table Out"=w423:variant)  [unwired: 6 in]
            n152 = Bundle By Name(cluster=w425, "TCP.Refs"=w424, "Addresses.LUT"=w423) -> (w422:T2)
          }
          frame "UI.Disable" {
            n153 = Unbundle By Name(w434) -> ("UI.Refs"=w440:T8)
            n154 = call "Workspace.UI.DisableState.Set.vi"("error in (no error)"=w437, "Enable?"=FALSE, "UI.Refs"=w440) -> ("error out"=w436:errorcluster, "UI.Refs out"=w439:T8)  [unwired: 7 in]
            n155 = Bundle By Name(cluster=w434, "UI.Refs"=w439) -> (w435:T2)
          }
          frame "UI.Enable" {
            n156 = Unbundle By Name(w442) -> ("UI.Refs"=w448:T8)
            n157 = call "Workspace.UI.DisableState.Set.vi"("error in (no error)"=w445, "Enable?"=TRUE, "UI.Refs"=w448) -> ("error out"=w444:errorcluster, "UI.Refs out"=w447:T8)  [unwired: 7 in]
            n158 = Bundle By Name(cluster=w442, "UI.Refs"=w447) -> (w443:T2)
          }
          frame Default {
            n159 = Concatenate Strings(w451, " is not a valid command." ("string")) -> (w450:string)
            n160 = One Button Dialog(message=w450) -> ()  [unwired: 1 in, 1 out]
          }
        }
      }
      frame Error {
        n161 = call <vilib>:"Simple Error Handler.vi"("error in (no error)"=w461) -> ("error out"=w460:errorcluster)  [unwired: 4 in, 4 out]
        n162 = call <vilib>:"Clear Errors.vi"("error in (no error)"=w460) -> ("error out"=w459:errorcluster)  [unwired: 5 in, 1 out]
      }
    }
  }
  n163 = Unbundle By Name(w22) -> ("NIVS.Workspace"=w17:T6, "NIVS.State.Refs"=w18:T7, "State.Notifier"=w20:refnum<user-event>, "LaunchConfig.Ref"=w21:refnum<user-event>, "Events.Refs"=w19:T12, "TCP.Refs"=w16:T4, "Errors.Q"=w13:refnum<queue>)
  n164 = flat-sequence {
    tunnel: w21 -> [w475]
    tunnel: w20 -> [w474]
    tunnel: w19 -> [w473]
    tunnel: w18 -> [w472]
    tunnel: w17 -> [w471]
    tunnel: w16 -> [w465]
    tunnel: w13 -> [w462]
    tunnel: [w470] -> w11
    tunnel: [w469] -> w10
    tunnel: [w468] -> w9
    tunnel: [w467] -> w8
    tunnel: [w466] -> w7
    tunnel: [w464] -> w6
    tunnel: [w463] -> w5
    tunnel: w11 -> [_]
    tunnel: w10 -> [_]
    tunnel: w9 -> [_]
    tunnel: w8 -> [_]
    tunnel: w7 -> [_]
    tunnel: w6 -> [_]
    tunnel: w5 -> [_]
    tunnel: [w476] -> _
    frame #0 {
      n165 = call <vilib>:"NI VeriStand - Close Workspace Manager Reference.vi"("WorkspaceManager"=w471) -> ("error out"=w470:errorcluster)  [unwired: 10 in]
      n166 = call <vilib>:"NI VeriStand - Close Engine State Change Notification.vi"("SystemStateRefs"=w472) -> ("error out"=w469:errorcluster)  [unwired: 10 in]
      n167 = Destroy User Event(user event=w474) -> (error out=w468:errorcluster)  [unwired: 1 in]
      n168 = Destroy User Event(user event=w475) -> (error out=w467:errorcluster)  [unwired: 1 in]
      n169 = Unregister For Events(event registration refnum=w473) -> (error out=w466:errorcluster)  [unwired: 1 in]
      n170 = call "STM Close Connection.vi"("connection info"=w465) -> ("error out"=w464:errorcluster)  [unwired: 10 in]
      n171 = Release Queue(queue=w462) -> (error out=w463:errorcluster)  [unwired: 2 in, 2 out]
    }
    frame #1 {
      n172 = invoke class="VI" method="FP.Close"() -> (error out=w476:errorcluster)  [unwired: 3 in, 2 out]
    }
  }
